vi "Find_Closeest_Embedding_Idx.vi"(5 "Selected_Coreset_Element_Info":T1, 7 "Pixel_Thrshld(Custom)":sgl, 11 "Distance_From_Embedding":sgl[](array[numeric])) -> (3 "Closest_Samples":T4[](array[typedef]))   [LabVIEW 2020]
uses:
  Controls/Closest_Sample_Info.ctl
  <vilib>/Ngene/DeepLTK Anomaly Detection Addon/Toolkit/API/Controls/Feature_Coords(Idx,i,j).ctl
  Controls/Selected_Coreset_Elements_and_Dim_Stride_Info.ctl
  Controls/Dims(2D)ctl.ctl
  <vilib>/Ngene/DeepLTK Anomaly Detection Addon/Toolkit/DeepLTK_Anomaly_Detection_Addon.lvlib
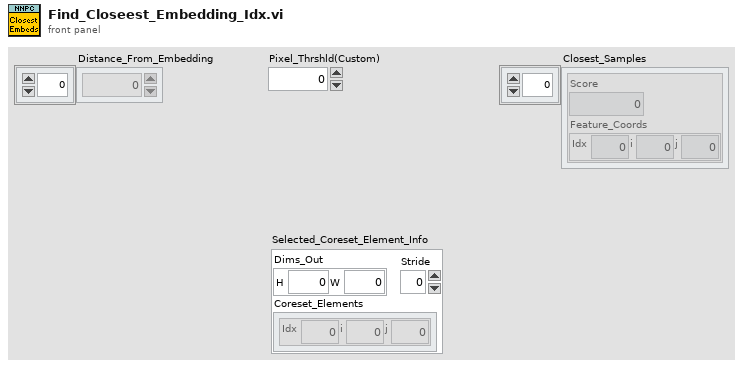
[diagram p1: front panel]
types:
  T1 = typedef "Selected_Coreset_Elements_and_Dim_Stride_Info.ctl" = cluster{"Dims_Out":T2, "Stride":i32, "Coreset_Elements":T3[]}
  T2 = typedef "Dims(2D)ctl.ctl" = cluster{"H":i32, "W":i32}
  T3 = typedef "DeepLTK_Anomaly_Detection_Addon.lvlib/Feature_Coords(Idx,i,j).ctl" = cluster{"Idx":i32, "i":i32, "j":i32}
  T4 = typedef "Closest_Sample_Info.ctl" = cluster{"Score":sgl, "Feature_Coords":T3}
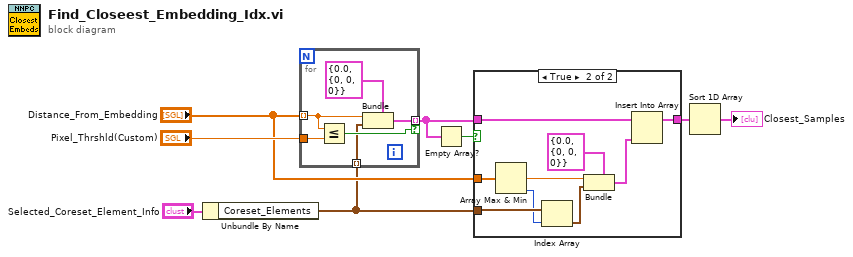
[diagram p0: block diagram]
diagram:
  n1 = Unbundle By Name("Selected_Coreset_Element_Info") -> ("Coreset_Elements"=w2:T3[])
  n2 = for {
    tunnel: "Pixel_Thrshld(Custom)" -> [w14]
    tunnel: "Distance_From_Embedding" -> [w13] mode=indexing
    tunnel: [w12] -> w4 mode=indexing if=w11
    tunnel: w2 -> [w10] mode=indexing
    n3 = Less Or Equal?(x=w13, y=w14) -> (x <= y?=w11:bool)
    n4 = Bundle(cluster=T4 {"Score"=0.0, "Feature_Coords"={"Idx"=0, "i"=0, "j"=0}}, "Score"=w13, "Feature_Coords"=w10) -> (w12:T4)
  }
  n5 = Empty Array?(array=w4) -> (empty?=w7:bool)
  n6 = case shown="True" w7 {
    tunnel: w4 -> [w15 w24]
    tunnel: [w15 w23] -> w6
    tunnel: "Distance_From_Embedding" -> [_ w22]
    tunnel: w2 -> [_ w20]
    frame False {
    }
    frame True {
      n7 = Array Max & Min(array=w22) -> (min value=w19:sgl, min index (indices)=w17:i32)  [unwired: 2 out]
      n8 = Index Array(array=w20, index=w17) -> (element=w18:T3)
      n9 = Bundle(cluster=T4 {"Score"=0.0, "Feature_Coords"={"Idx"=0, "i"=0, "j"=0}}, "Score"=w19, "Feature_Coords"=w18) -> (w21:T4)
      n10 = Insert Into Array(array=w24, new element=w21) -> (w23:T4[])  [unwired: 1 in]
    }
  }
  n11 = Sort 1D Array(array=w6) -> (sorted array=→"Closest_Samples":T4[])
